vi "貪食蛇.vi"() -> ()   [LabVIEW 2014]
uses:
  <vilib>/Utility/inputDevices.llb/keyboardAcquire.vi
  <vilib>/Utility/inputDevices.llb/closeKeyboard.vi
panel:
  out "Wall":bool[][](array[boolean])
  out "Map  Width 2":i32=25
  out "Map Length 2":i32=25
  out "Food":bool[][](array[boolean])
  out "difficulty add":dbl
  out "Restart":bool
  out "Original Position":i16[][](array[numeric])
  out "Condition":enum16{"TasteAwful", "Hurt", "GoGo"}(ring)
  in  "Level":dbl=1.0
  out "element":T1(ring)
  in  "Map  Width":i32=25
  in  "Map Length":i32=25
  out "Mood":bool
  in  "stop":bool
  out "Map":bool[][](array[boolean])
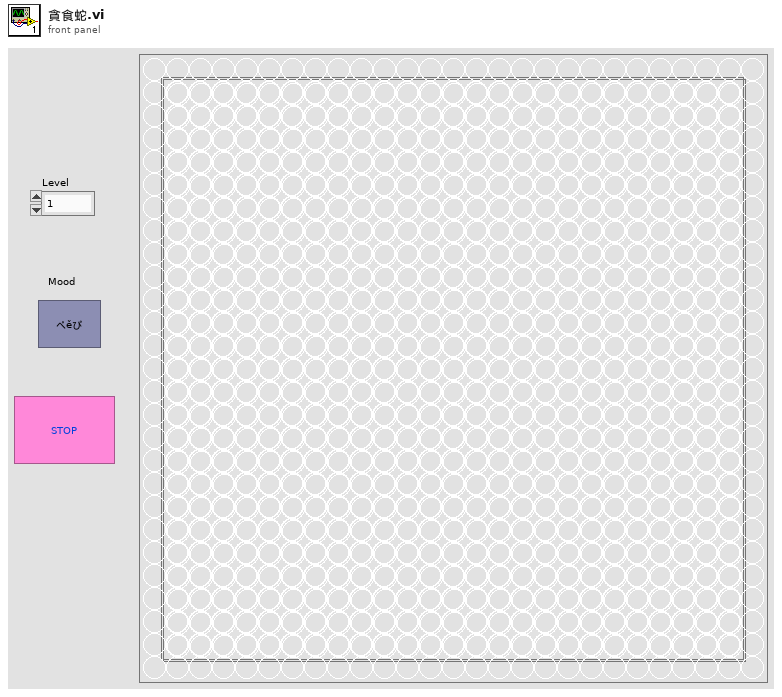
[diagram p1: front panel]
types:
  T1 = enum16{"0", "1", "2", "3", "4", "5", "6", "7", "8", "9", "A", "B", "C", "D", "E", "F", "G", "H", "I", "J", "K", "L", "M", "N", "O", "P", "Q", "R", "S", "T", "U", "V", "W", "X", "Y", "Z", "F1", "F2", "F3", "F4", "F5", "F6", "F7", "F8", "F9", "F10", "F11", "F12", "F13", "F14", "F15", "ADD", "BACK", "BACKSLASH", "CAPITAL", "COMMA", "DECIMAL", "DELETE", "DIVIDE", "DOWN", "END", "EQUALS", "ESCAPE", "GRAVE (`)", "HOME", "INSERT", "LBRACKET", "LCONTROL", "LEFT", "L ALT", "LSHIFT", "LWIN", "MINUS", "MULTIPLY", "NEXT", "NUMLOCK", "NUMPAD_0", "NUMPAD_1", "NUMPAD_2", "NUMPAD_3", "NUMPAD_4", "NUMPAD_5", "NUMPAD_6", "NUMPAD_7", "NUMPAD_8", "NUMPAD_9", "PAUSE", "PERIOD", "PRIOR (PG UP)", "RBRACKET", "RCONTROL", "RETURN", "RIGHT", "R ALT", "RSHIFT", "RWIN", "SCROLL", "SEMICOLON", "SLASH", "SPACE", "SUBTRACT", "TAB", "UP", "ENTER (num pad)", "' (quote)"}
  T2 = enum16{"0", "1", "2", "3", "4", "5", "6", "7", "8", "9", "A", "B", "C", "D", "E", "F", "G", "H", "I", "J", "K", "L", "M", "N", "O", "P", "Q", "R", "S", "T", "U", "V", "W", "X", "Y", "Z", "F1", "F2", "F3", "F4", "F5", "F6", "F7", "F8", "F9", "F10", "F11", "F12", "F13", "F14", "F15", "ADD", "BACK", "BACKSLASH", "CAPITAL", "COMMA", "DECIMAL", "DELETE", "DIVIDE", "DOWN", "END", "EQUALS", "ESCAPE", "GRAVE (`)", "HOME", "INSERT", "LBRACKET", "LCONTROL", "LEFT", "L ALT", "LSHIFT", "LWIN", "MINUS", "MULTIPLY", "NEXT", "NUMLOCK", "NUMPAD_0", "NUMPAD_1", "NUMPAD_2", "NUMPAD_3", "NUMPAD_4", "NUMPAD_5", "NUMPAD_6", "NUMPAD_7", "NUMPAD_8", "NUMPAD_9", "PAUSE", "PERIOD", "PRIOR (PG UP)", "RBRACKET", "RCONTROL", "RETURN", "RIGHT", "R ALT", "RSHIFT", "RWIN", "SCROLL", "SEMICOLON", "SLASH", "SPACE", "SUBTRACT", "TAB", "UP", "ENTER (num pad)", "' (quote)"}[]
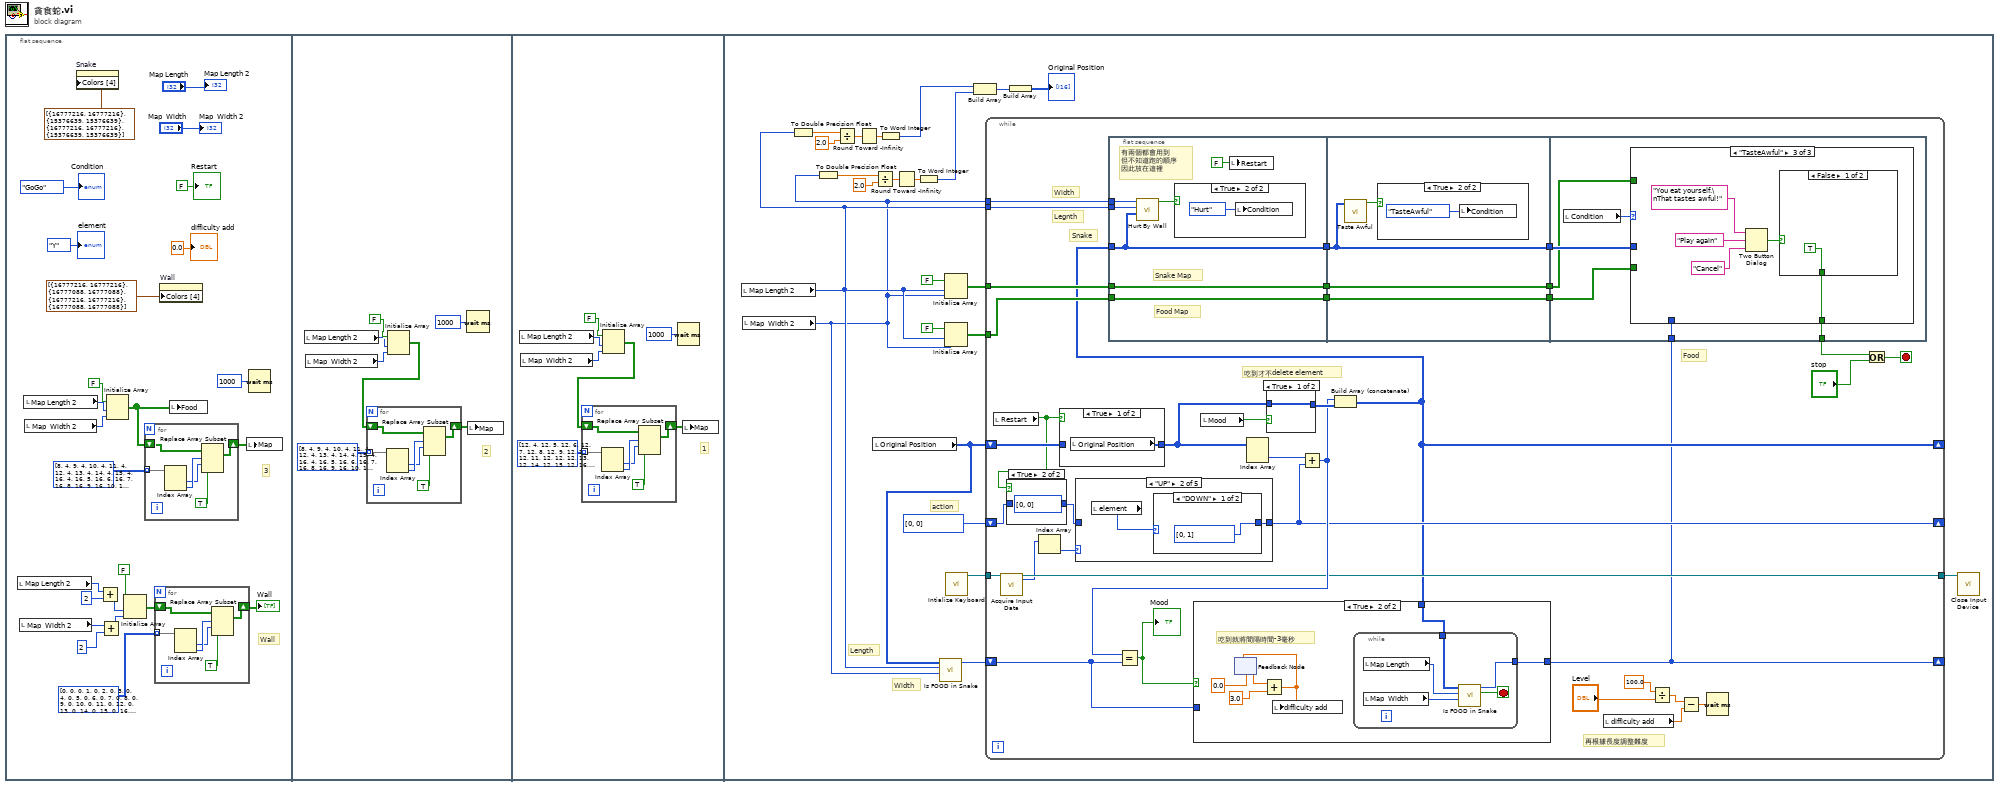
[diagram p0: block diagram]
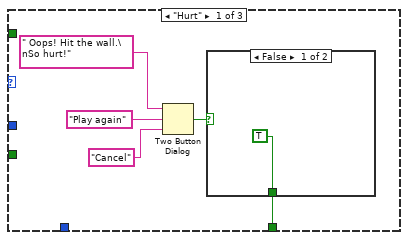
[diagram p6: hidden frame]
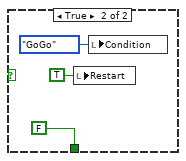
[diagram p7: hidden frame]
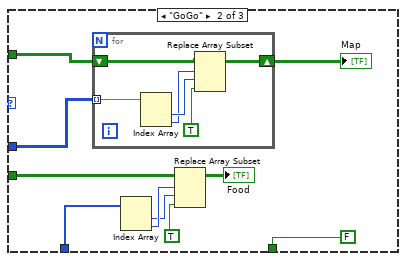
[diagram p8: hidden frame]
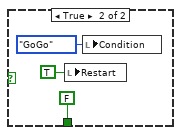
[diagram p9: hidden frame]
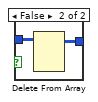
[diagram p11: hidden frame]
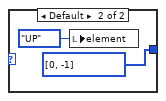
[diagram p13: hidden frame]
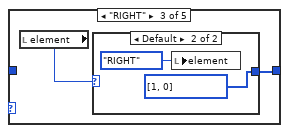
[diagram p14: hidden frame]
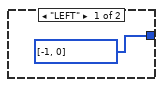
[diagram p15: hidden frame]
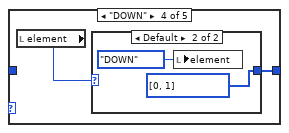
[diagram p16: hidden frame]
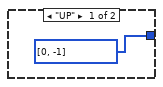
[diagram p17: hidden frame]
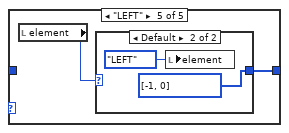
[diagram p18: hidden frame]
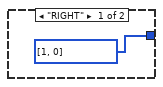
[diagram p19: hidden frame]
diagram:
  n1 = flat-sequence {
    frame #0 {
      # "Wall"
      # "3"
      n2 = local read "Map Length 2"() -> (w10:i32)
      n3 = local read "Map  Width 2"() -> (w8:i32)
      n4 = local read "Map Length 2"() -> (w15:i32)
      n5 = local read "Map  Width 2"() -> (w14:i32)
      n6 = property on="Snake" class="Bool (strict)"("Colors [4]"=cluster{u32, u32}[] [{16777216, 16777216}, {15376639, 15376639}, {16777216, 16777216}, {15376639, 15376639}]) -> ()  [unwired: 2 in, 2 out]
      n7 = Add(x=w10, y=2) -> (x+y=w5:i32)
      n8 = Add(x=w8, y=2) -> (x+y=w6:i32)
      n9 = Initialize Array(FALSE, w15, w14) -> (w12:bool[][])
      n10 = Initialize Array(FALSE, w5, w6) -> (w4:bool[][])
      n11 = for {
        shift-right: [w32] -> w17
        shift-left: w12 -> [w34]
        tunnel: i32[][] [[8, 4], [9, 4], [10, 4], [11, 4], [12, 4], [13, 4], [14, 4], [15, 4], [16, 4], [16, 5], [16, 6], [16, 7], [16, 8], [16, 9], [16, 10], [16, 11], [8, 12], [9, 12], [10, 12], [11, 12], [12, 12], [13, 12], [14, 12], [15, 12], [16, 12], [16, 13], [16, 14], [16, 15], [16, 16], [16, 17], [16, 18], [16, 19], [8, 20], [9, 20], [10, 20], [11, 20], [12, 20], [13, 20], [14, 20], [15, 20], [16, 20]] ("appended array") -> [w37] mode=indexing
        n12 = Index Array(array=w37) -> (element #1=w35:i32, element #2=w36:i32)  [unwired: 2 in]
        n13 = Replace Array Subset(array=w34, new element=TRUE ("new element/subarray"), index (row)=w36, index (col)=w35) -> (w32:bool[][])
      }
      n14 = for {
        shift-right: [w26] -> w2
        shift-left: w4 -> [w28]
        tunnel: i32[][] [[0, 0], [0, 1], [0, 2], [0, 3], [0, 4], [0, 5], [0, 6], [0, 7], [0, 8], [0, 9], [0, 10], [0, 11], [0, 12], [0, 13], [0, 14], [0, 15], [0, 16], [0, 17], [0, 18], [0, 19], [0, 20], [0, 21], [0, 22], [0, 23], [0, 24], [0, 25], [0, 26], [0, 0], [26, 0], [26, 1], [26, 2], [26, 3], [26, 4], [26, 5], [26, 6], [26, 7], [26, 8], [26, 9], [26, 10], [26, 11], [26, 12], [26, 13], [26, 14], [26, 15], [26, 16], [26, 17], [26, 18], [26, 19], [26, 20], [26, 21], [26, 22], [26, 23], [26, 24], [26, 25], [26, 26], [0, 0], [1, 0], [2, 0], [3, 0], [4, 0], [5, 0], [6, 0], [7, 0], [8, 0], [9, 0], [10, 0], [11, 0], [12, 0], [13, 0], [14, 0], [15, 0], [16, 0], [17, 0], [18, 0], [19, 0], [20, 0], [21, 0], [22, 0], [23, 0], [24, 0], [25, 0], [0, 0], [1, 26], [2, 26], [3, 26], [4, 26], [5, 26], [6, 26], [7, 26], [8, 26], [9, 26], [10, 26], [11, 26], [12, 26], [13, 26], [14, 26], [15, 26], [16, 26], [17, 26], [18, 26], [19, 26], [20, 26], [21, 26], [22, 26], [23, 26], [24, 26], [25, 26], [0, 0]] ("appended array") -> [w31] mode=indexing
        n15 = Index Array(array=w31) -> (element #1=w29:i32, element #2=w30:i32)  [unwired: 2 in]
        n16 = Replace Array Subset(array=w28, new element=TRUE ("new element/subarray"), index (row)=w30, index (col)=w29) -> (w26:bool[][])
      }
      "Wall" <- w2
      n17 = property on="Wall" class="Bool (strict)"("Colors [4]"=cluster{u32, u32}[] [{16777216, 16777216}, {16777088, 16777088}, {16777216, 16777216}, {16777088, 16777088}]) -> ()  [unwired: 2 in, 2 out]
      n18 = local write "Food"(w12) -> ()
      n19 = local write "Map"(w17) -> ()
      n20 = Wait (ms)(milliseconds to wait=u32 1000) -> ()  [unwired: 1 out]
      "element" <- T1."Y" ("element")
      "Condition" <- enum16{"TasteAwful", "Hurt", "GoGo"}."GoGo"
      "Restart" <- FALSE ("Restart")
      "difficulty add" <- 0.0
      "Map Length 2" <- "Map Length"
      "Map  Width 2" <- "Map  Width"
    }
    frame #1 {
      # "2"
      n21 = local read "Map Length 2"() -> (w40:i32)
      n22 = local read "Map  Width 2"() -> (w41:i32)
      n23 = Initialize Array(FALSE, w40, w41) -> (w39:bool[][])
      n24 = for {
        shift-right: [w45] -> w38
        shift-left: w39 -> [w47]
        tunnel: i32[][] [[8, 4], [9, 4], [10, 4], [11, 4], [12, 4], [13, 4], [14, 4], [15, 4], [16, 4], [16, 5], [16, 6], [16, 7], [16, 8], [16, 9], [16, 10], [16, 11], [8, 12], [9, 12], [10, 12], [11, 12], [12, 12], [13, 12], [14, 12], [15, 12], [16, 12], [8, 13], [8, 14], [8, 15], [8, 16], [8, 17], [8, 18], [8, 19], [8, 20], [9, 20], [10, 20], [11, 20], [12, 20], [13, 20], [14, 20], [15, 20], [16, 20]] ("appended array") -> [w50] mode=indexing
        n25 = Index Array(array=w50) -> (element #1=w48:i32, element #2=w49:i32)  [unwired: 2 in]
        n26 = Replace Array Subset(array=w47, new element=TRUE ("new element/subarray"), index (row)=w49, index (col)=w48) -> (w45:bool[][])
      }
      n27 = Wait (ms)(milliseconds to wait=u32 1000) -> ()  [unwired: 1 out]
      n28 = local write "Map"(w38) -> ()
    }
    frame #2 {
      # "1"
      n29 = local read "Map Length 2"() -> (w54:i32)
      n30 = local read "Map  Width 2"() -> (w53:i32)
      n31 = Initialize Array(FALSE, w54, w53) -> (w55:bool[][])
      n32 = for {
        shift-right: [w58] -> w56
        shift-left: w55 -> [w60]
        tunnel: i32[][] [[12, 4], [12, 5], [12, 6], [12, 7], [12, 8], [12, 9], [12, 10], [12, 11], [12, 12], [12, 13], [12, 14], [12, 15], [12, 16], [12, 17], [12, 18], [12, 19], [12, 20]] ("appended array") -> [w63] mode=indexing
        n33 = Index Array(array=w63) -> (element #1=w61:i32, element #2=w62:i32)  [unwired: 2 in]
        n34 = Replace Array Subset(array=w60, new element=TRUE ("new element/subarray"), index (row)=w62, index (col)=w61) -> (w58:bool[][])
      }
      n35 = Wait (ms)(milliseconds to wait=u32 1000) -> ()  [unwired: 1 out]
      n36 = local write "Map"(w56) -> ()
    }
    frame #3 {
      # "Length"
      # "Width"
      # "action"
      n37 = local read "Map Length 2"() -> (w65:i32)
      n38 = local read "Map  Width 2"() -> (w64:i32)
      n39 = To Double Precision Float(number=w65) -> (double precision float=w71:dbl)
      n40 = To Double Precision Float(number=w64) -> (double precision float=w70:dbl)
      n41 = Divide(x=w71, y=2.0) -> (x/y=w80:dbl)
      n42 = Round Toward -Infinity(1:w80) -> (0:w79:dbl)
      n43 = local read "Original Position"() -> (w68:i16[][])
      n44 = Divide(x=w70, y=2.0) -> (x/y=w74:dbl)
      n45 = To Word Integer(number=w79) -> (16bit integer=w78:i16)
      n46 = Round Toward -Infinity(1:w74) -> (0:w73:dbl)
      n47 = To Word Integer(number=w73) -> (16bit integer=w72:i16)
      n48 = call "Is FOOD in Snake.vi"("Map width"=w64, "Map Length"=w65, "Snake Position"=w68) -> ("Food Position"=w69:i32[])  [unwired: 7 in, 1 out]
      n49 = Initialize Array(FALSE, w65, w64) -> (w85:bool[][])
      n50 = Initialize Array(FALSE, w65, w64) -> (w66:bool[][])
      n51 = call <vilib>:"Intialize Keyboard.vi"() -> ("device ID"=w84:refnum<k1>)  [unwired: 10 in, 1 out]
      n52 = Build Array(w78, w72) -> (w77:i16[])
      n53 = while {
        tunnel: w85 -> [w111]
        tunnel: w84 -> [w94]
        tunnel: [w95] -> w83
        shift-right: [w89] -> _
        shift-left: w68 -> [w105]
        shift-right: [w102] -> _
        shift-left: i32[] [0, 0] -> [w101]
        shift-right: [w88] -> _
        shift-left: w69 -> [w119]
        tunnel: w64 -> [w115]
        tunnel: w65 -> [w114]
        tunnel: w66 -> [w92]
        stop <- w106 stop-if-true
        # "Legnth"
        # "Width"
        # "Snake"
        # "Food"
        # "再根據長度調整難度"
        # "吃到才不delete element"
        n54 = local read "Restart"() -> (w99:bool)
        n55 = call-poly <vilib>:"Acquire Input Data.vi"("device ID"=w94) -> ("device ID"=w95:refnum<k1>, "keys pressed"=w93:T2)  [unwired: 16 in, 1 out]
        n56 = case shown="True" w99 {
          tunnel: w101 -> [w123 _]
          tunnel: [w123 i32[] [0, 0]] -> w100
          frame False {
          }
          frame True {
          }
        }
        n57 = Index Array(array=w93) -> (element=w118:T1)  [unwired: 1 in]
        n58 = case shown="True" w99 {
          tunnel: w105 -> [_ w126]
          tunnel: [w125 w126] -> w104
          frame True {
            n59 = local read "Original Position"() -> (w125:i16[][])
          }
          frame False {
          }
        }
        n60 = case shown="\"UP\"" w118 {
          tunnel: w100 -> [w195 _ _ _ _]
          tunnel: [w195 w197 w202 w206 w211] -> w102
          frame Default {
          }
          frame "UP" {
            n61 = local read "element"() -> (w196:T1)
            n62 = case shown="\"DOWN\"" w196 {
              tunnel: [i32[] [0, 1] i32[] [0, -1]] -> w197
              frame "DOWN" {
              }
              frame Default {
                n63 = local write "element"(T1."UP" ("element")) -> ()
              }
            }
          }
          frame "RIGHT" {
            n64 = local read "element"() -> (w201:T1)
            n65 = case shown="Default" w201 {
              tunnel: [i32[] [-1, 0] i32[] [1, 0]] -> w202
              frame "LEFT" {
              }
              frame Default {
                n66 = local write "element"(T1."RIGHT" ("element")) -> ()
              }
            }
          }
          frame "DOWN" {
            n67 = local read "element"() -> (w207:T1)
            n68 = case shown="Default" w207 {
              tunnel: [i32[] [0, -1] i32[] [0, 1]] -> w206
              frame "UP" {
              }
              frame Default {
                n69 = local write "element"(T1."DOWN" ("element")) -> ()
              }
            }
          }
          frame "LEFT" {
            n70 = local read "element"() -> (w212:T1)
            n71 = case shown="Default" w212 {
              tunnel: [i32[] [1, 0] i32[] [-1, 0]] -> w211
              frame "RIGHT" {
              }
              frame Default {
                n72 = local write "element"(T1."LEFT" ("element")) -> ()
              }
            }
          }
        }
        n73 = flat-sequence {
          tunnel: w115 -> [w132]
          tunnel: w114 -> [w131]
          tunnel: w89 -> [w130]
          tunnel: [w130] -> w113
          tunnel: w111 -> [w129]
          tunnel: [w129] -> w110
          tunnel: w92 -> [w128]
          tunnel: [w128] -> w90
          tunnel: w113 -> [w137]
          tunnel: [w137] -> w112
          tunnel: w110 -> [w136]
          tunnel: [w136] -> w109
          tunnel: [w135] -> w91
          tunnel: w90 -> [w135]
          tunnel: w112 -> [w144]
          tunnel: w109 -> [w143]
          tunnel: [w142] -> w103
          tunnel: w91 -> [w140]
          tunnel: w88 -> [w141]
          frame #0 {
            # "Snake Map"
            # "Food Map"
            # "有兩個都會用到\n但不知道跑的順序\n因此放在這裡"
            n74 = call "Hurt By Wall.vi"("Array"=w130, "Map Length"=w131, "Map  Width"=w132) -> ("Boolean"=w133:bool)  [unwired: 8 in]
            n75 = case shown="True" w133 {
              frame False {
              }
              frame True {
                n76 = local write "Condition"(enum16{"TasteAwful", "Hurt", "GoGo"}."Hurt" ("Condition")) -> ()
              }
            }
            n77 = local write "Restart"(FALSE ("Restart")) -> ()
          }
          frame #1 {
            n78 = call "Taste Awful.vi"("Array"=w137) -> ("logical AND"=w138:bool)  [unwired: 10 in]
            n79 = case shown="True" w138 {
              frame False {
              }
              frame True {
                n80 = local write "Condition"(enum16{"TasteAwful", "Hurt", "GoGo"}."TasteAwful" ("Condition")) -> ()
              }
            }
          }
          frame #2 {
            n81 = local read "Condition"() -> (w145:enum16{"TasteAwful", "Hurt", "GoGo"})
            n82 = case shown="\"TasteAwful\"" w145 {
              tunnel: w143 -> [_ w164 _]
              tunnel: w144 -> [_ w163 _]
              tunnel: [w146 FALSE w171] -> w142
              tunnel: w141 -> [_ w158 _]
              tunnel: w140 -> [_ w157 _]
              frame "Hurt" {
                n83 = Two Button Dialog(message=" Oops! Hit the wall.\nSo hurt!", 1:"Cancel" ("F button name (\"Cancel\")"), 2:"Play again" ("T button name (\"OK\")")) -> (T button?=w147:bool)
                n84 = case shown="False" w147 {
                  tunnel: [TRUE FALSE] -> w146
                  frame False {
                  }
                  frame True {
                    n85 = local write "Restart"(TRUE ("Restart")) -> ()
                    n86 = local write "Condition"(enum16{"TasteAwful", "Hurt", "GoGo"}."GoGo" ("Condition")) -> ()
                  }
                }
              }
              frame "GoGo" {
                n87 = for {
                  shift-right: [w169] -> w155
                  shift-left: w164 -> [w170]
                  tunnel: w163 -> [w168] mode=indexing
                  n88 = Index Array(array=w168) -> (element #1=w167:i32, element #2=w166:i32)  [unwired: 2 in]
                  n89 = Replace Array Subset(array=w170, new element=TRUE ("new element/subarray"), index (row)=w166, index (col)=w167) -> (w169:bool[][])
                }
                "Map" <- w155
                n90 = Index Array(array=w158) -> (element #1=w159:i32, element #2=w160:i32)  [unwired: 2 in]
                n91 = Replace Array Subset(array=w157, new element=TRUE ("new element/subarray"), index (row)=w160, index (col)=w159) -> (→"Food":bool[][])
              }
              frame "TasteAwful" {
                n92 = Two Button Dialog(message="You eat yourself.\nThat tastes awful!", 1:"Cancel" ("F button name (\"Cancel\")"), 2:"Play again" ("T button name (\"OK\")")) -> (T button?=w172:bool)
                n93 = case shown="False" w172 {
                  tunnel: [TRUE FALSE] -> w171
                  frame False {
                  }
                  frame True {
                    n94 = local write "Restart"(TRUE ("Restart")) -> ()
                    n95 = local write "Condition"(enum16{"TasteAwful", "Hurt", "GoGo"}."GoGo" ("Condition")) -> ()
                  }
                }
              }
            }
          }
        }
        n96 = local read "Mood"() -> (w120:bool)
        n97 = Index Array(array=w104) -> (element=w121:i32[])  [unwired: 2 in]
        n98 = case shown="True" w120 {
          tunnel: [w192 w194] -> w122
          tunnel: w104 -> [w192 w193]
          frame True {
          }
          frame False {
            n99 = Delete From Array(array=w193) -> (array with subset deleted=w194:i32[][])  [unwired: 3 in, 1 out]
          }
        }
        n100 = Add(x=w121, y=w102) -> (x+y=w108:i32[])
        n101 = Equal?(x=w108, y=w119) -> (x = y?=w107:bool)
        "Mood" <- w107
        n102 = Build Array (concatenate)(w108, w122) -> (w89:i32[][])
        n103 = case shown="True" w107 {
          tunnel: w89 -> [_ w186]
          tunnel: [w180 w185] -> w88
          tunnel: w119 -> [w180 _]
          frame False {
          }
          frame True {
            # "吃到就將間隔時間-3毫秒"
            n104 = feedback #1(0.0) -> (w183:dbl)
            n105 = Add(x=w183, y=3.0) -> (x+y=w181:dbl)
            n106 = feedback-in #1(w181) -> ()
            n107 = local write "difficulty add"(w181) -> ()
            n108 = while {
              tunnel: w186 -> [w191]
              tunnel: [w189] -> w185
              stop <- w190 stop-if-true
              n109 = local read "Map Length"() -> (w188:i32)
              n110 = local read "Map  Width"() -> (w187:i32)
              n111 = call "Is FOOD in Snake.vi"("Map width"=w187, "Map Length"=w188, "Snake Position"=w191) -> ("Boolean"=w190:bool, "Food Position"=w189:i32[])  [unwired: 7 in]
            }
          }
        }
        n112 = local read "difficulty add"() -> (w96:dbl)
        n113 = Divide(x=100.0 ("millisecond multiple"), y="Level") -> (x/y=w98:dbl)
        n114 = Subtract(x=w98, y=w96) -> (x-y=w97:dbl)
        n115 = Wait (ms)(milliseconds to wait=w97) -> ()  [unwired: 1 out]
        n116 = Or(x=w103, y="stop") -> (x .or. y?=w106:bool)
      }
      n117 = Build Array(w77) -> (→"Original Position":i16[][])
      n118 = call-poly <vilib>:"Close Input Device.vi"("device ID"=w83) -> ()  [unwired: 9 in, 1 out]
    }
  }
